vi "sub_Array to Index.vi"(10 "索引 (行)":i32, 11 "All Random Array":dbl[][](array[numeric])) -> (0 "y offset new":dbl, 1 "x offset new":dbl, 2 "y amp. new":dbl, 3 "x amp. new":dbl, 6 "Row Number":i32)   [LabVIEW 2015]
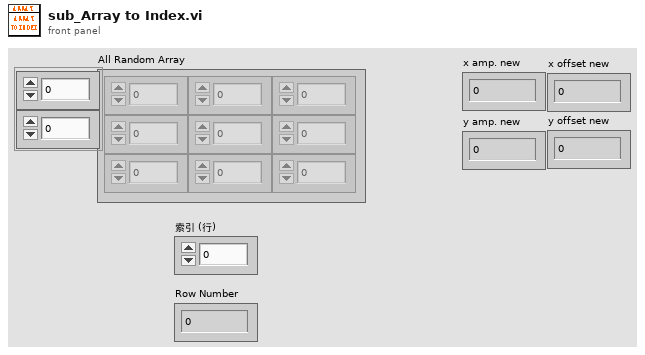
[diagram p1: front panel]
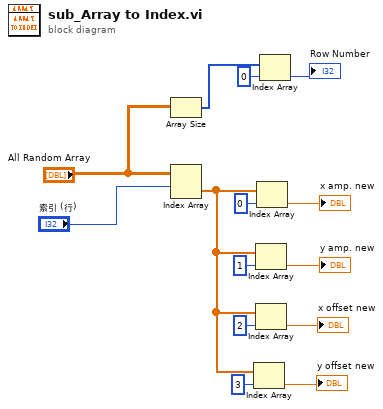
[diagram p0: block diagram]
diagram:
  n1 = Array Size(array="All Random Array") -> (size(s)=w2:i32[])
  n2 = Index Array(array="All Random Array", index (row)="索引 (行)") -> (element=w9:dbl[])  [unwired: 1 in]
  n3 = Index Array(array=w9, index=3 ("索引")) -> (element=→"y offset new":dbl)
  n4 = Index Array(array=w9, index=1 ("索引")) -> (element=→"y amp. new":dbl)
  n5 = Index Array(array=w9, index=2 ("索引")) -> (element=→"x offset new":dbl)
  n6 = Index Array(array=w9, index=0 ("索引")) -> (element=→"x amp. new":dbl)
  n7 = Index Array(array=w2, index=0 ("索引")) -> (element=→"Row Number":i32)
